vi "FFT Output_Ping Pong Data between BRAM.vi"(5 "Read Count":u16, 7 "Write Count":u16, 8 "Input Valid":bool, 10 "Bank1 Data":T1, 11 "Bank0 Data":T2) -> (0 "Read Valid":bool, 2 "Address1. Element Out":u16, 3 "Address0. Element Out":u16, 4 "Read Address 1":u16, 6 "Read Address 0":u16)   [LabVIEW 2011]
doc: "This VI does ping pong between two BRAM blocks\n\n<b> Latency = 3 Ticks </b>"
uses:
  <vilib>/rvi/FXPMathLib/basic elements/FxpDiscreteDelay/XNode/nifxpmath_DiscreteDelay.xnode
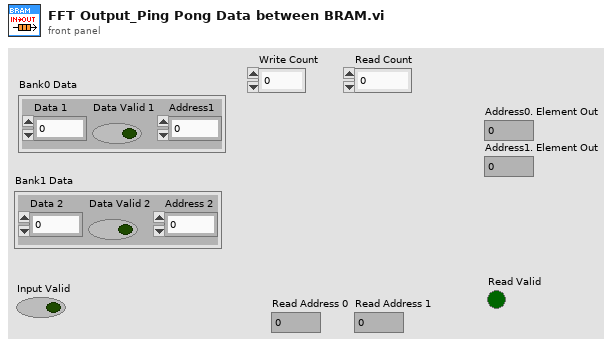
[diagram p1: front panel]
types:
  T1 = cluster{"Data 2":u64, "Data Valid 2":bool, "Address 2":u16}
  T2 = cluster{"Data 1":u64, "Data Valid 1":bool, "Address1":u16}
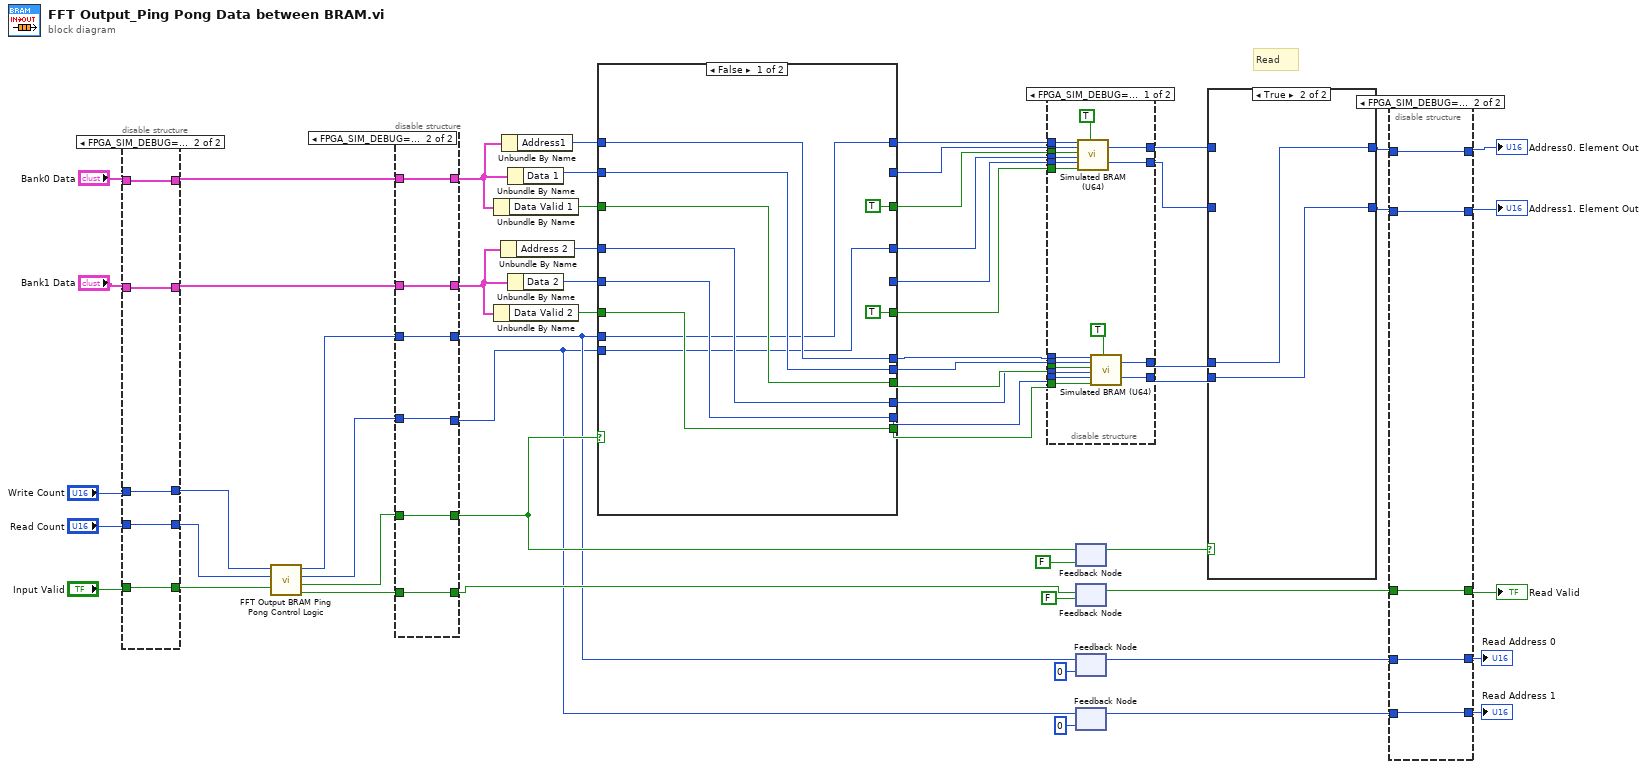
[diagram p0: block diagram]
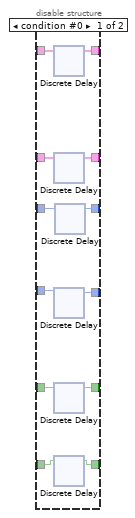
[diagram p2: hidden frame]
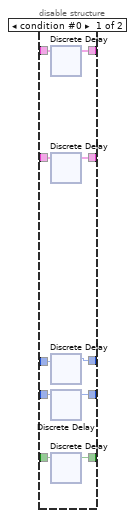
[diagram p3: hidden frame]
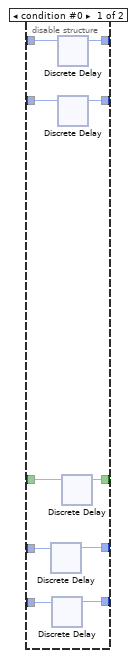
[diagram p4: hidden frame]
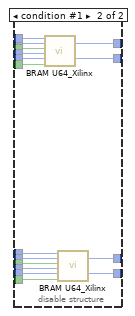
[diagram p5: hidden frame]
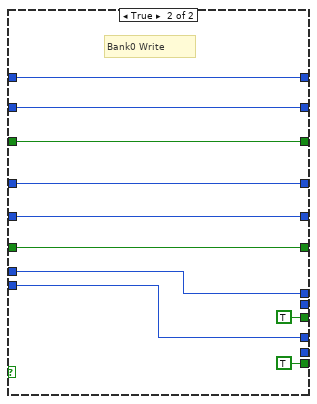
[diagram p7: hidden frame]
diagram:
  # "Read"
  n1 = disable-structure shown="FPGA_SIM_DEBUG==TRUE" {
    disable-tunnel: "Bank0 Data" -> [w67 w72]
    disable-tunnel: "Bank1 Data" -> [w66 w71]
    disable-tunnel: "Input Valid" -> [w65 w68]
    disable-tunnel: "Write Count" -> [w64 w70]
    disable-tunnel: "Read Count" -> [w63 w69]
    disable-tunnel: [w62 w72] -> w25
    disable-tunnel: [w61 w71] -> w24
    disable-tunnel: [w60 w68] -> w23
    disable-tunnel: [w59 w70] -> w19
    disable-tunnel: [w58 w69] -> w18
    frame condition #0 {
      n2 = xnode "Discrete Delay"("D"=w67) -> ("Q"=w62:T2)
      n3 = xnode "Discrete Delay"("D"=w66) -> ("Q"=w61:T1)
      n4 = xnode "Discrete Delay"("D"=w64) -> ("Q"=w59:u16)
      n5 = xnode "Discrete Delay"("D"=w63) -> ("Q"=w58:u16)
      n6 = xnode "Discrete Delay"("D"=w65) -> ("Q"=w60:bool)
    }
    frame condition #1 (active) {
    }
  }
  n7 = call <userlib>:"FFT Output BRAM Ping Pong Control Logic.vi"("Input Valid"=w23, "Read Count"=w18, "Write Count"=w19) -> ("Read Valid"=w32:bool, "BRAM Bank0 Write?"=w13:bool, "Read Address 2"=w12:u16, "Read Address1"=w11:u16)  [unwired: 5 in]
  n8 = disable-structure shown="FPGA_SIM_DEBUG==TRUE" {
    disable-tunnel: w32 -> [w84 w85]
    disable-tunnel: w12 -> [w83 w87]
    disable-tunnel: w13 -> [w82 w86]
    disable-tunnel: w25 -> [w81 w90]
    disable-tunnel: w24 -> [w80 w89]
    disable-tunnel: [w79 w87] -> w1
    disable-tunnel: [w78 w89] -> w17
    disable-tunnel: [w77 w90] -> w16
    disable-tunnel: [w76 w86] -> w15
    disable-tunnel: [w75 w85] -> w14
    disable-tunnel: w11 -> [w74 w88]
    disable-tunnel: [w73 w88] -> w2
    frame condition #0 {
      n9 = xnode "Discrete Delay"("D"=w81) -> ("Q"=w77:T2)
      n10 = xnode "Discrete Delay"("D"=w80) -> ("Q"=w78:T1)
      n11 = xnode "Discrete Delay"("D"=w83) -> ("Q"=w79:u16)
      n12 = xnode "Discrete Delay"("D"=w82) -> ("Q"=w76:bool)
      n13 = xnode "Discrete Delay"("D"=w84) -> ("Q"=w75:bool)
      n14 = xnode "Discrete Delay"("D"=w74) -> ("Q"=w73:u16)
    }
    frame condition #1 (active) {
    }
  }
  n15 = Unbundle By Name(w16) -> ("Data Valid 1"=w46:bool)
  n16 = Unbundle By Name(w17) -> ("Data Valid 2"=w39:bool)
  n17 = Unbundle By Name(w17) -> ("Address 2"=w43:u16)
  n18 = Unbundle By Name(w16) -> ("Address1"=w49:u16)
  n19 = Unbundle By Name(w16) -> ("Data 1"=w50:u64)
  n20 = Unbundle By Name(w17) -> ("Data 2"=w42:u64)
  n21 = case shown="False" w15 {
    tunnel: w50 -> [w99 w109]
    tunnel: w46 -> [w98 w108]
    tunnel: [_ w109] -> w57
    tunnel: w49 -> [w100 w110]
    tunnel: [w92 w110] -> w48
    tunnel: [TRUE ("Data Valid 1") w108] -> w44
    tunnel: w43 -> [w97 w107]
    tunnel: [w91 w107] -> w41
    tunnel: w42 -> [w96 w106]
    tunnel: [_ w106] -> w40
    tunnel: w39 -> [w95 w105]
    tunnel: [TRUE ("Data Valid 2") w105] -> w38
    tunnel: [w100 w102] -> w10
    tunnel: [w99 _] -> w37
    tunnel: [w98 TRUE ("Data Valid 1")] -> w36
    tunnel: [w97 w101] -> w9
    tunnel: [w96 _] -> w35
    tunnel: [w95 TRUE ("Data Valid 2")] -> w34
    tunnel: w2 -> [w92 w102]
    tunnel: w1 -> [w91 w101]
    frame False {
    }
    frame True {
      # "Bank0 Write"
    }
  }
  n22 = disable-structure shown="FPGA_SIM_DEBUG==TRUE" {
    disable-tunnel: w57 -> [w128 w144]
    disable-tunnel: [w127 w143] -> w56
    disable-tunnel: [w126 w142] -> w55
    disable-tunnel: [w125 w141] -> w54
    disable-tunnel: [w124 w140] -> w53
    disable-tunnel: w48 -> [w123 w139]
    disable-tunnel: w44 -> [w122 w138]
    disable-tunnel: w41 -> [w121 w137]
    disable-tunnel: w40 -> [w120 w136]
    disable-tunnel: w38 -> [w119 w135]
    disable-tunnel: w10 -> [w118 w134]
    disable-tunnel: w37 -> [w117 w133]
    disable-tunnel: w36 -> [w116 w132]
    disable-tunnel: w9 -> [w115 w131]
    disable-tunnel: w35 -> [w114 w130]
    disable-tunnel: w34 -> [w113 w129]
    frame condition #0 (active) {
      n23 = call <userlib>:"Simulated BRAM (U64).vi"("Address 0"=w123, "Address0.Element In"=w128, "Address 0 Write"=w122, "Address 1"=w121, "Address1.Element In"=w120, "Address 1 Write"=w119, "Read Before Write?"=TRUE) -> ("Address0. Element Out"=w127:u64, "Address1. Element Out"=w126:u64)  [unwired: 10 in, 1 out]
      n24 = call <userlib>:"Simulated BRAM (U64).vi"("Address 0"=w118, "Address0.Element In"=w117, "Address 0 Write"=w116, "Address 1"=w115, "Address1.Element In"=w114, "Address 1 Write"=w113, "Read Before Write?"=TRUE) -> ("Address0. Element Out"=w125:u64, "Address1. Element Out"=w124:u64)  [unwired: 10 in, 1 out]
    }
    frame condition #1 {
      n25 = call <userlib>:"BRAM U64_Xilinx.vi"("Address 0"=w139, "Address0.Data"=w144, "Address0.Write?"=w138, "Address 1"=w137, "Address 1.Data"=w136, "Address1 Write?"=w135) -> ("Address 0.Element"=w143:u64, "Address 1.Element"=w142:u64)  [unwired: 12 in]
      n26 = call <userlib>:"BRAM U64_Xilinx.vi"("Address 0"=w134, "Address0.Data"=w133, "Address0.Write?"=w132, "Address 1"=w131, "Address 1.Data"=w130, "Address1 Write?"=w129) -> ("Address 0.Element"=w141:u64, "Address 1.Element"=w140:u64)  [unwired: 12 in]
    }
  }
  n27 = feedback-in #1(w15) -> ()
  n28 = feedback #1(FALSE ("BRAM Bank0 Write?")) -> (w27:bool)
  n29 = feedback-in #2(w14) -> ()
  n30 = feedback #2(FALSE ("Read Valid")) -> (w29:bool)
  n31 = feedback-in #3(w2) -> ()
  n32 = feedback #3(u16 0 ("Read Address1")) -> (w8:u16)
  n33 = feedback-in #4(w1) -> ()
  n34 = feedback #4(u16 0 ("Read Address 2")) -> (w7:u16)
  n35 = case shown="True" w27 {
    tunnel: w56 -> [w146 _]
    tunnel: w55 -> [w145 _]
    tunnel: w54 -> [_ w148]
    tunnel: w53 -> [_ w147]
    tunnel: [w146 w148] -> w52
    tunnel: [w145 w147] -> w51
    frame False {
    }
    frame True {
    }
  }
  n36 = disable-structure shown="FPGA_SIM_DEBUG==TRUE" {
    disable-tunnel: w52 -> [w158 w163]
    disable-tunnel: w51 -> [w157 w162]
    disable-tunnel: w29 -> [w156 w161]
    disable-tunnel: [w155 w161] -> w22
    disable-tunnel: [w154 w162] -> w21
    disable-tunnel: [w153 w163] -> w20
    disable-tunnel: w8 -> [w152 w160]
    disable-tunnel: w7 -> [w151 w159]
    disable-tunnel: [w150 w160] -> w6
    disable-tunnel: [w149 w159] -> w5
    frame condition #0 {
      n37 = xnode "Discrete Delay"("D"=w152) -> ("Q"=w150:u16)
      n38 = xnode "Discrete Delay"("D"=w151) -> ("Q"=w149:u16)
      n39 = xnode "Discrete Delay"("D"=w158) -> ("Q"=w153:u64)
      n40 = xnode "Discrete Delay"("D"=w157) -> ("Q"=w154:u64)
      n41 = xnode "Discrete Delay"("D"=w156) -> ("Q"=w155:bool)
    }
    frame condition #1 (active) {
    }
  }
  "Address0. Element Out" <- w20
  "Address1. Element Out" <- w21
  "Read Valid" <- w22
  "Read Address 0" <- w6
  "Read Address 1" <- w5
